vi "Testbench for Servo.vi"() -> ()   [LabVIEW 2011]
doc: "Elizabeth Mahon and Olli Gallitz\n\nGenerates string for servo contoller and sends it down to the FPGA and servo controller."
uses:
  <vilib>/FPGAPlugInAG/cRIO-9113/niLvFpga_Close_cRIO-9113.vi
  <vilib>/rvi/interface/nirviCloseFPGA/nirviCloseFPGA.xnode
  FPGA Bitfiles/SailBot_FPGATarget_3AFPGAReadFromFI_976E4797.lvbitx
  1,3 A-Competition Platform/1,3 A Code/3A FPGA ReadFromFIFOPort4.vi
panel:
  in  "Winch":i32
  in  "Rudder":dbl
  in  "stop":bool
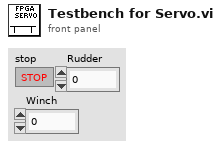
[diagram p1: front panel]
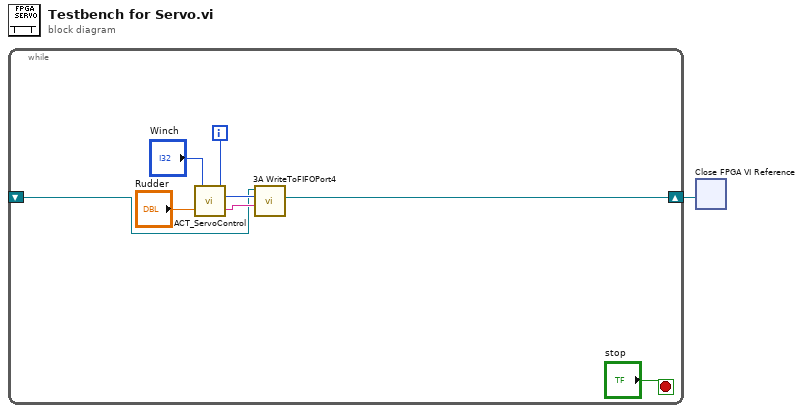
[diagram p0: block diagram]
diagram:
  n1 = while {
    shift-right: [w3] -> w1
    shift-left: _ -> [w2]
    i -> [w5]
    stop <- "stop" stop-if-true
    n2 = call "ACT_ServoControl.vi"("y 2"="Rudder", "y"="Winch") -> ("String"=w6:string)  [unwired: 1 in]
    n3 = call "3A WriteToFIFOPort4.vi"("String"=w6, "loop#"=w5, "FPGA VI Reference Out"=w2) -> ("FPGA VI Reference Out 2"=w3:refnum<k20>)  [unwired: 8 in]
  }
  n4 = xnode "Close FPGA VI Reference"("FPGA VI Reference In"=w1) -> ()  [unwired: 1 in, 1 out]
